vi "GDSLvClass_MethodOverrideCheck.vi"(8 "error in (no error)":errorcluster, 10 "ProjectItem Refnum":refnum<vi>, 11 "LVClassLibrary in":refnum<vi>) -> (0 "error out":errorcluster, 2 "GetMustOverride":bool, 3 "LVClassLibrary out":refnum<vi>)   [LabVIEW 2020]
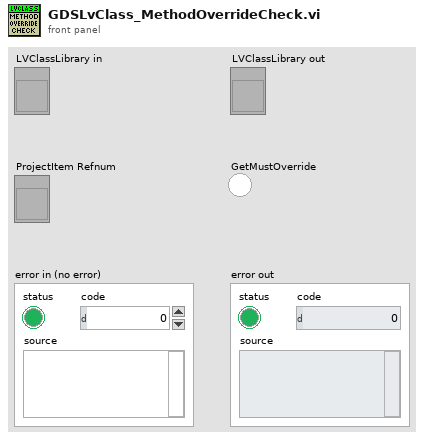
[diagram p1: front panel]
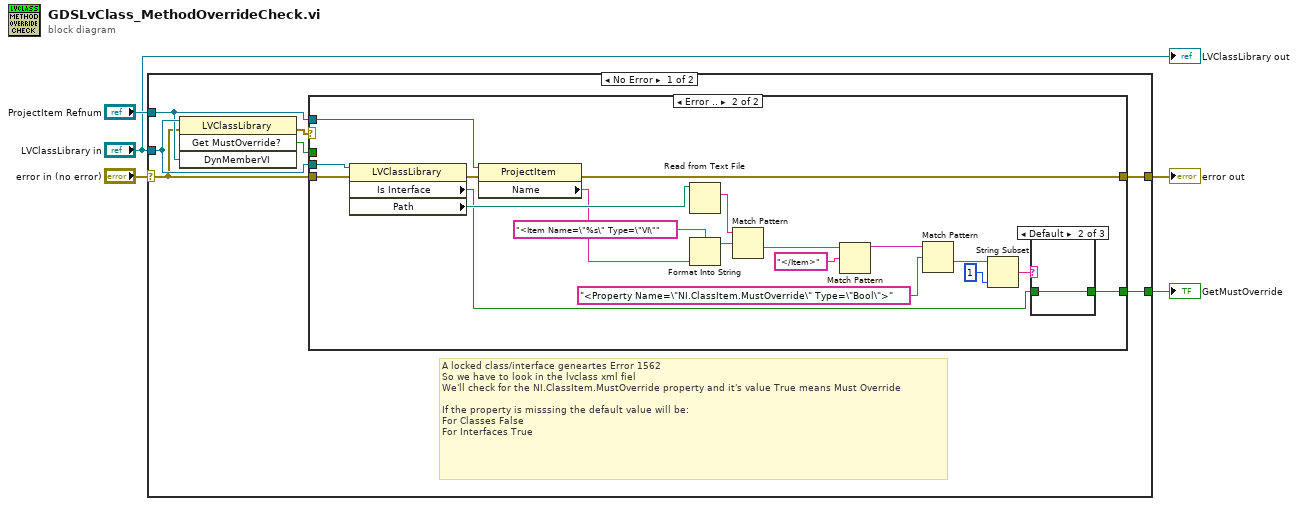
[diagram p0: block diagram]
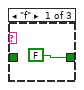
[diagram p3: hidden frame]
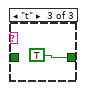
[diagram p4: hidden frame]
diagram:
  n1 = case shown="No Error" "error in (no error)" {
    selector: "error in (no error)" -> [w6 w37]
    tunnel: [w9 w37] -> w5
    tunnel: "ProjectItem Refnum" -> [w7 _]
    tunnel: "LVClassLibrary in" -> [w8 _]
    tunnel: [w10 _] -> w1
    frame No Error {
      # "A locked class/interface geneartes Error 1562\nSo we have to look in the lvclass xml fiel\nWe'll check for the NI.ClassItem.MustOverride property and it's value True means Must Override\n\nIf the property is misssing the default value will be:\nFor Classes False\nFor Interfaces True"
      n2 = invoke class="LVClassLibrary" method="Get MustOverride?"(reference=w8, error in=w6, "DynMemberVI"=w7) -> (error out=w12:errorcluster, "GetMustOverride"=w11:bool)  [unwired: 1 in, 2 out]
      n3 = case shown="Error .." w12 {
        selector: w12 -> [w13 _]
        tunnel: w11 -> [w14 _]
        tunnel: [w14 w20] -> w10
        tunnel: [w13 w16] -> w9
        tunnel: w8 -> [_ w33]
        tunnel: w7 -> [_ w29]
        tunnel: w6 -> [_ w18]
        frame No Error {
        }
        frame Error {
          n4 = property class="LVClassLibrary"(reference=w33, error in=w18) -> (error out=w17:errorcluster, "Is Interface"=w19:bool, "Path"=w32:path)  [unwired: 1 out]
          n5 = property class="ProjectItem"(reference=w29, error in=w17) -> (error out=w16:errorcluster, "Name"=w28:string)  [unwired: 1 out]
          n6 = Read from Text File(file (use dialog)=w32) -> (text=w31:string)  [unwired: 3 in, 3 out]
          n7 = Format Into String(format string="<Item Name=\"%s\" Type=\"VI\"", w28) -> (resulting string=w27:string)  [unwired: 2 in, 1 out]
          n8 = Match Pattern(string=w31, regular expression=w27) -> (after substring=w26:string)  [unwired: 1 in, 3 out]
          n9 = Match Pattern(string=w26, regular expression="</Item>") -> (before substring=w24:string)  [unwired: 1 in, 3 out]
          n10 = Match Pattern(string=w24, regular expression="<Property Name=\"NI.ClassItem.MustOverride\" Type=\"Bool\">") -> (after substring=w15:string)  [unwired: 1 in, 3 out]
          n11 = String Subset(string=w15, length (rest)=1 ("length (rest)")) -> (substring=w21:string)  [unwired: 1 in]
          n12 = case shown="Default" w21 {
            tunnel: [FALSE w35 TRUE] -> w20
            tunnel: w19 -> [_ w35 _]
            frame "f" {
            }
            frame Default {
            }
            frame "t" {
            }
          }
        }
      }
    }
    frame Error {
    }
  }
  "error out" <- w5
  "GetMustOverride" <- w1
  "LVClassLibrary out" <- "LVClassLibrary in"
